vi "PeriodicFilter-Check Speed.vi"(7 "seconds since 1Jan1904":timestamp, 8 "Settings":T3={"threashold(#/s)"=1.0, "Check Peroid(s)"=1.0}, 9 "Parameter":string, 10 "index":i32, 11 "data in":T1 {"LastCheckT" format="%<%.3X>T"}) -> (0 "over threashold?":bool, 1 "new filtered Item":bool, 3 "data out":T1 {"LastCheckT" format="%<%.3X>T"})   [LabVIEW 2017, in "Communicable State Machine.lvlib"]
uses:
  Communicable State Machine.lvlib
  Periodic String Filter Data.ctl
  Periodic String Filter Info.ctl
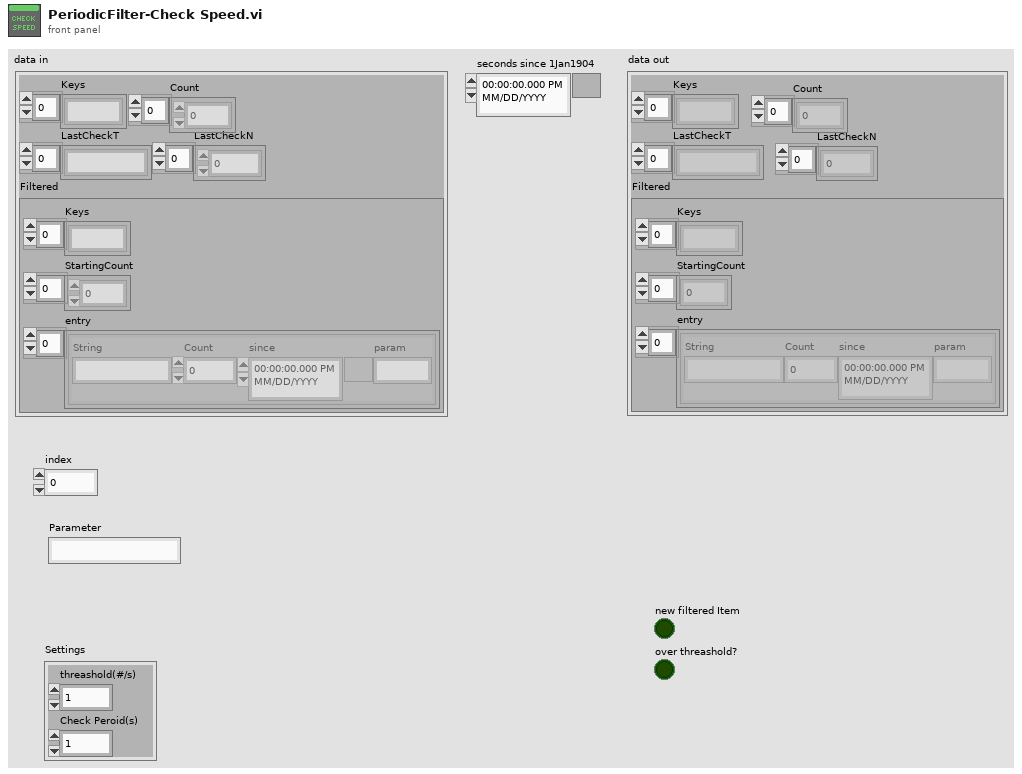
[diagram p1: front panel]
types:
  T1 = typedef "Communicable State Machine.lvlib/Periodic String Filter Data.ctl" = cluster{"Keys":string[], "Count":i64[], "LastCheckT":timestamp[], "LastCheckN":i64[], "Filtered":cluster{"Keys":string[], "StartingCount":i64[], "entry":T2[]}}
  T2 = typedef "Communicable State Machine.lvlib/Periodic String Filter Info.ctl" = cluster{"String":string, "Count":i64, "since":timestamp, "param":string}
  T3 = cluster{"threashold(#/s)":dbl, "Check Peroid(s)":dbl}
  T4 = cluster{"Keys":string[], "StartingCount":i64[], "entry":T2[]}
  T5 = cluster{"Input String 2":string, i64, "seconds since 1Jan1904":timestamp, "Parameter":string}
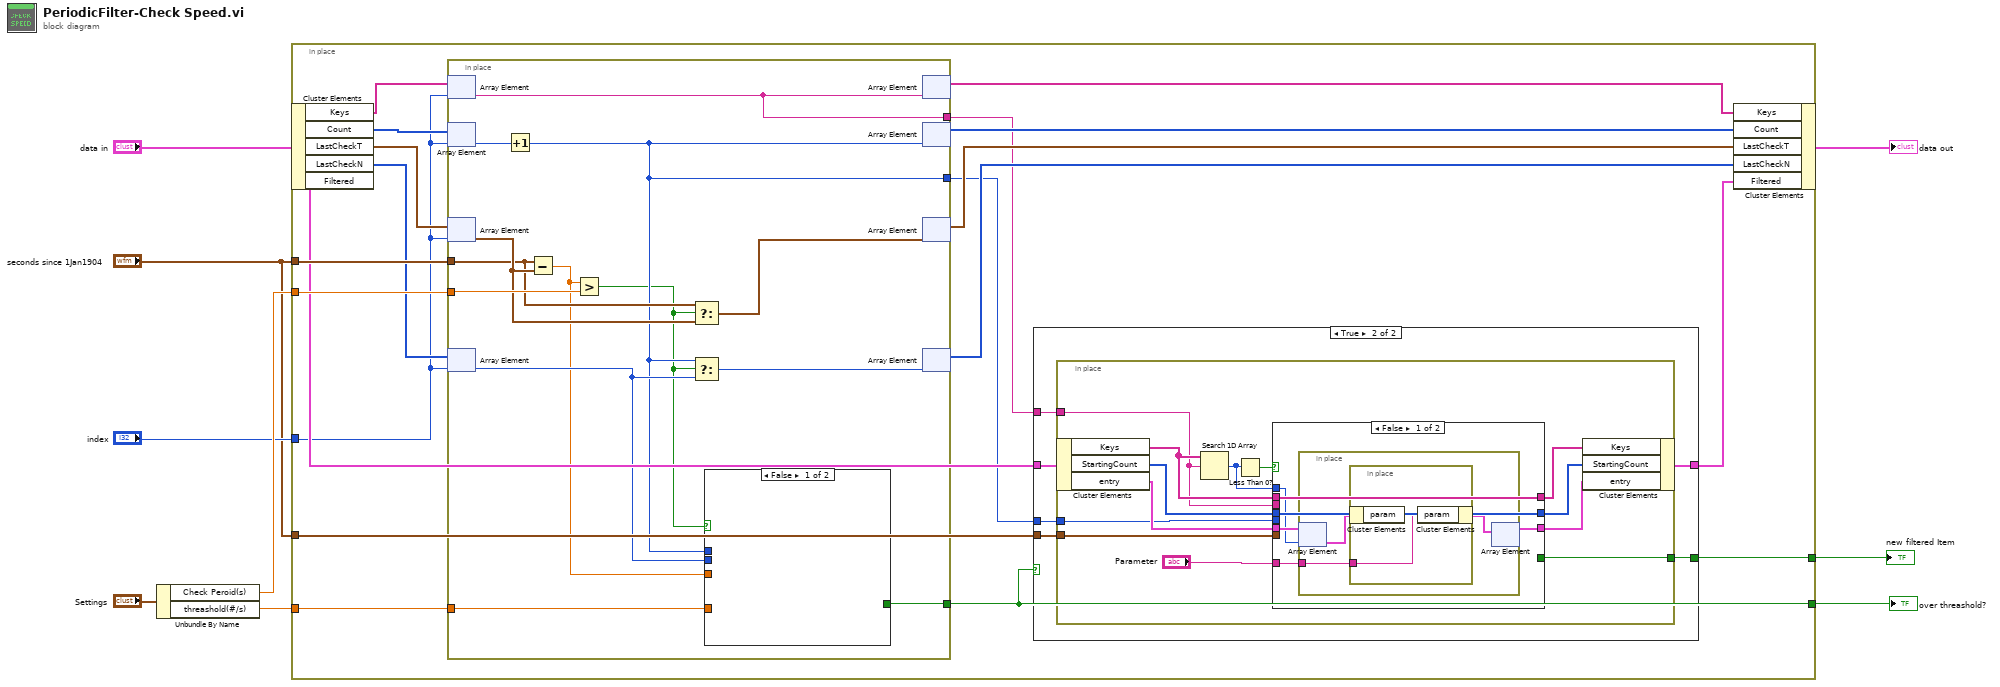
[diagram p0: block diagram]
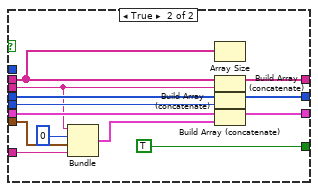
[diagram p3: hidden frame]
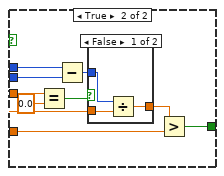
[diagram p4: hidden frame]
diagram:
  n1 = Unbundle By Name("Settings") -> ("Check Peroid(s)"=w9:dbl, "threashold(#/s)"=w8:dbl)
  n2 = in-place "In Place Element Structure" {
    in-place-border: w9 -> [w28]
    in-place-border: "index" -> [w16]
    in-place-border: w8 -> [w27]
    in-place-border: [w11] -> w6
    in-place-border: "seconds since 1Jan1904" -> [w26]
    in-place-border: "seconds since 1Jan1904" -> [w18]
    in-place-border: [w10] -> w1
    n3 = in-place-cluster #1("data in") -> ("Keys"=w17:string[], "Count"=w25:i64[], "LastCheckT"=w22:timestamp[], "LastCheckN"=w23:i64[], "Filtered"=w19:T4)
    n4 = in-place {
      in-place-border: w26 -> [w81]
      in-place-border: w28 -> [w83]
      in-place-border: w27 -> [w77]
      in-place-border: [w76] -> w11
      in-place-border: [w75] -> w12
      in-place-border: [w74] -> w15
      n5 = in-place-array #2(w17, w16) -> (w74:string)
      n6 = in-place-array #3(w25, w16) -> (w84:i64)
      n7 = in-place-array #4(w22, w16) -> (w82:timestamp)
      n8 = in-place-array #5(w23, w16) -> (w78:i64)
      n9 = Increment(x=w84) -> (x+1=w75:i64)
      n10 = Subtract(x=w81, y=w82) -> (x-y=w73:dbl)
      n11 = Greater?(x=w73, y=w83) -> (0:w72:bool)
      n12 = Select(t=w81, s=w72, f=w82) -> (s? t:f=w79:timestamp)
      n13 = Select(t=w75, s=w72, f=w78) -> (s? t:f=w80:i64)
      n14 = case shown="False" w72 {
        tunnel: w78 -> [_ w91]
        tunnel: w77 -> [_ w90]
        tunnel: [_ w89] -> w76
        tunnel: w75 -> [_ w88]
        tunnel: w73 -> [_ w87]
        frame False {
        }
        frame True {
          n15 = Equal?(x=w87, y=0.0) -> (x = y?=w85:bool)
          n16 = Subtract(x=w88, y=w91) -> (x-y=w92:i64)
          n17 = case shown="False" w85 {
            tunnel: [w96 _] -> w93
            tunnel: w92 -> [w95 _]
            tunnel: w87 -> [w94 _]
            frame False {
              n18 = Divide(x=w95, y=w94) -> (x/y=w96:dbl)
            }
            frame True {
            }
          }
          n19 = Greater?(x=w93, y=w90) -> (0:w89:bool)
        }
      }
      n20 = in-place-array #2(w74) -> (w13:string[])  [unwired: 1 out]
      n21 = in-place-array #3(w75) -> (w24:i64[])  [unwired: 1 out]
      n22 = in-place-array #4(w79) -> (w21:timestamp[])  [unwired: 1 out]
      n23 = in-place-array #5(w80) -> (w20:i64[])  [unwired: 1 out]
    }
    n24 = case shown="True" w11 {
      tunnel: w19 -> [w29 w35]
      tunnel: w18 -> [_ w34]
      tunnel: w15 -> [_ w33]
      tunnel: [w29 w32] -> w14
      tunnel: w12 -> [_ w31]
      tunnel: [_ w30] -> w10
      frame False {
      }
      frame True {
        n25 = in-place {
          in-place-border: w34 -> [w40]
          in-place-border: w33 -> [w39]
          in-place-border: w31 -> [w38]
          in-place-border: [w37] -> w30
          n26 = in-place-cluster #6(w35) -> ("Keys"=w46:string[], "StartingCount"=w44:i64[], "entry"=w45:T2[])
          n27 = Search 1D Array(1D array=w46, element=w39) -> (index of element=w47:i32)  [unwired: 1 in]
          n28 = Less Than 0?(x=w47) -> (x < 0?=w48:bool)
          n29 = case shown="False" w48 {
            tunnel: w46 -> [w54 w70]
            tunnel: w39 -> [_ w64]
            tunnel: [w54 w71] -> w43
            tunnel: w47 -> [w50 _]
            tunnel: w44 -> [w53 w69]
            tunnel: [w53 w68] -> w42
            tunnel: w45 -> [w52 w67]
            tunnel: w40 -> [_ w63]
            tunnel: [w51 w66] -> w41
            tunnel: w38 -> [_ w65]
            tunnel: [_ TRUE] -> w37
            tunnel: "Parameter" -> [w49 w59]
            frame False {
              n30 = in-place {
                in-place-border: w49 -> [w55]
                n31 = in-place-array #7(w52, w50) -> (w57:T2)
                n32 = in-place {
                  in-place-border: w55 -> [w58]
                  n33 = in-place-cluster #8(w57) -> ()  [unwired: 1 out]
                  n34 = in-place-cluster #8("param"=w58) -> (w56:T2)
                }
                n35 = in-place-array #7(w56) -> (w51:T2[])  [unwired: 1 out]
              }
            }
            frame True {
              n36 = Bundle("Input String 2"=w64, i64 0, "seconds since 1Jan1904"=w63, "Parameter"=w59) -> (w61:T5)  [unwired: 1 in]
              n37 = Array Size(array=w70) -> ()  [unwired: 1 out]
              n38 = Build Array (concatenate)(w70, w64) -> (w71:string[])
              n39 = Build Array (concatenate)(w69, w65) -> (w68:i64[])
              n40 = Build Array (concatenate)(w67, w61) -> (w66:T2[])
            }
          }
          n41 = in-place-cluster #6("Keys"=w43, "StartingCount"=w42, "entry"=w41) -> (w32:T4)
        }
      }
    }
    n42 = in-place-cluster #1("Keys"=w13, "Count"=w24, "LastCheckT"=w21, "LastCheckN"=w20, "Filtered"=w14) -> (→"data out":T1)
  }
  "over threashold?" <- w6
  "new filtered Item" <- w1
